vi "simple test.vi"() -> ()   [LabVIEW 2009]
uses:
  <vilib>/rvi/interface/nirviOpenFPGA/nirviOpenFPGA.xnode
  fpgaserialreadwrite_8.6/fpgaserialreadwrite_8.6_update/FPGA Bitfiles/FPGA RS232.lvproj_FPGA Target 2_RS422 chip test.vi.lvbitx
  <vilib>/FPGAPlugInAG/sbRIO-9642/nirviIntfOpen_sbRIO-9642.vi
  <vilib>/rvi/interface/nirviReadWriteControl/nirviReadWriteControl.xnode
  <vilib>/Utility/error.llb/Error Cluster From Error Code.vi
  <vilib>/rvi/errors/niLvFpgaAdjustHostInterfaceError.vi
  <vilib>/rvi/interface/common/niFpgaNodeNameForErrorReporting.ctl
  <vilib>/rvi/errors/niLvFpgaWhatHappensToTopLevelVI.ctl
  <vilib>/rvi/interface/nirviCloseFPGA/nirviCloseFPGA.xnode
  <vilib>/FPGAPlugInAG/sbRIO-9642/nirviIntfClose_sbRIO-9642.vi
  <vilib>/userDefined/High Color/nirio_resource_hc.ctl
  NiRioSrv.dll
panel:
  in  "stop":bool
  out "Waveform Chart":i16(graph)
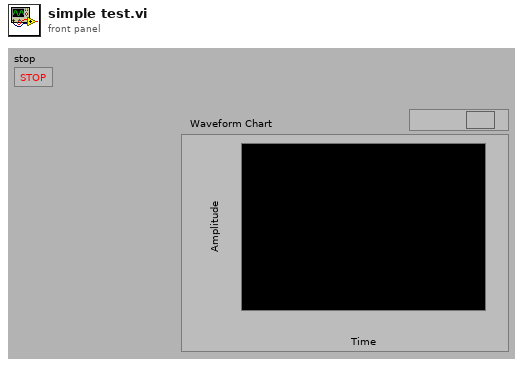
[diagram p1: front panel]
types:
  T1 = typedef "niFpgaNodeNameForErrorReporting.ctl" = enum16{"Open FPGA VI Reference", "Read/Write Control", "Invoke Method: Abort", "Invoke Method: Acknowledge IRQ", "Invoke Method: Download", "Invoke Method: FIFO.Configure", "Invoke Method: FIFO.Read", "Invoke Method: FIFO.Start", "Invoke Method: FIFO.Stop", "Invoke Method: FIFO.Write", "Invoke Method: Reset", "Invoke Method: Run", "Invoke Method: Wait on IRQ", "Close FPGA VI Reference"}
  T2 = typedef "niLvFpgaWhatHappensToTopLevelVI.ctl" = enum16{"top level VI scripted behind XNode", "top level VI inlined behind XNode"}
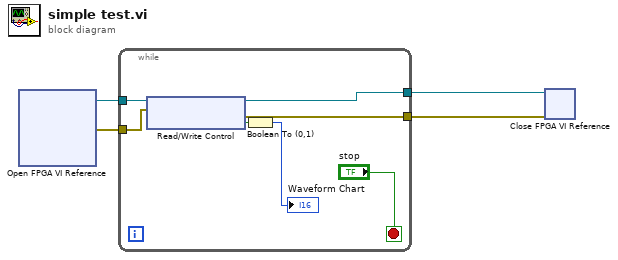
[diagram p0: block diagram]
diagram:
  n1 = xnode "Open FPGA VI Reference"() -> ("FPGA VI Reference Out"=w4:refnum<k20>, "error out"=w3:errorcluster)  [unwired: 2 in]
  n2 = while {
    tunnel: w4 -> [w11]
    tunnel: w3 -> [w10]
    tunnel: [w9] -> w2
    tunnel: [w8] -> w1
    stop <- "stop" stop-if-true
    n3 = xnode "Read/Write Control"("FPGA VI Reference In"=w11, "error in"=w10) -> ("FPGA VI Reference Out"=w8:refnum<k20>, "error out"=w9:errorcluster, "'RS422' Recieve"=w7:bool)
    n4 = Boolean To (0,1)(Boolean=w7) -> (0, 1=→"Waveform Chart":i16)
  }
  n5 = xnode "Close FPGA VI Reference"("FPGA VI Reference In"=w1, "error in"=w2) -> ()  [unwired: 1 out]
